vi "Settings for BLE.vi"(0 "Sp_Id_Arr":string[](array[string]), 5 "Ex_Mod_IDs":string[](array[string]), 7 "Est Thresh Val":dbl, 9 "Threshold Value Analysis":bool) -> (4 "Thresh Val":dbl[](array[numeric]), 6 "Index":i32[](array[numeric]), 8 "No of I/ps":i32)   [LabVIEW 2014]
panel:
  in  "Enter Threshold Values":string[][](array[string])=[["GFP", "5", "55", "34"], ["LacI", "10", "55", "34"], ["TetR", "10", "55", "34"]]
  in  "Select Output Specie":u16(ring)=1 items=["GFP", "P1", "P2"]
  in  "OK":bool caption="OK1"
  out "Output Sp":string[](array[string])
  # "Logic Verification Settings"
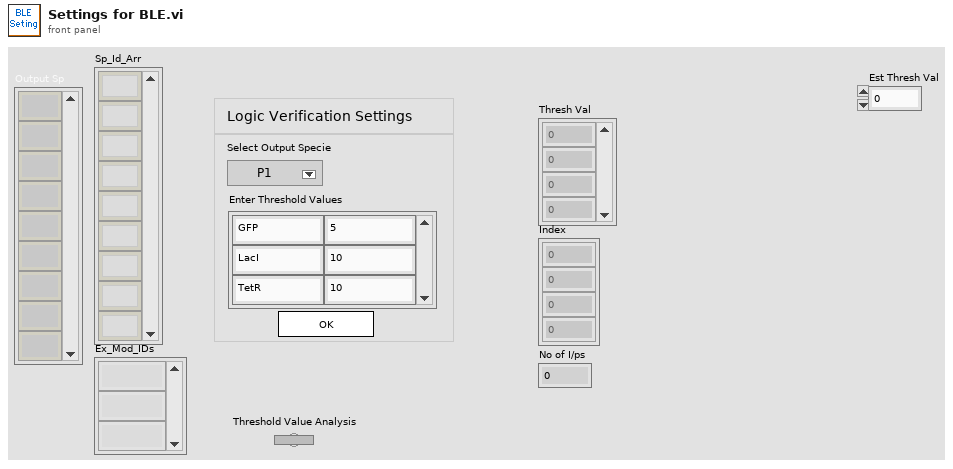
[diagram p1: front panel]
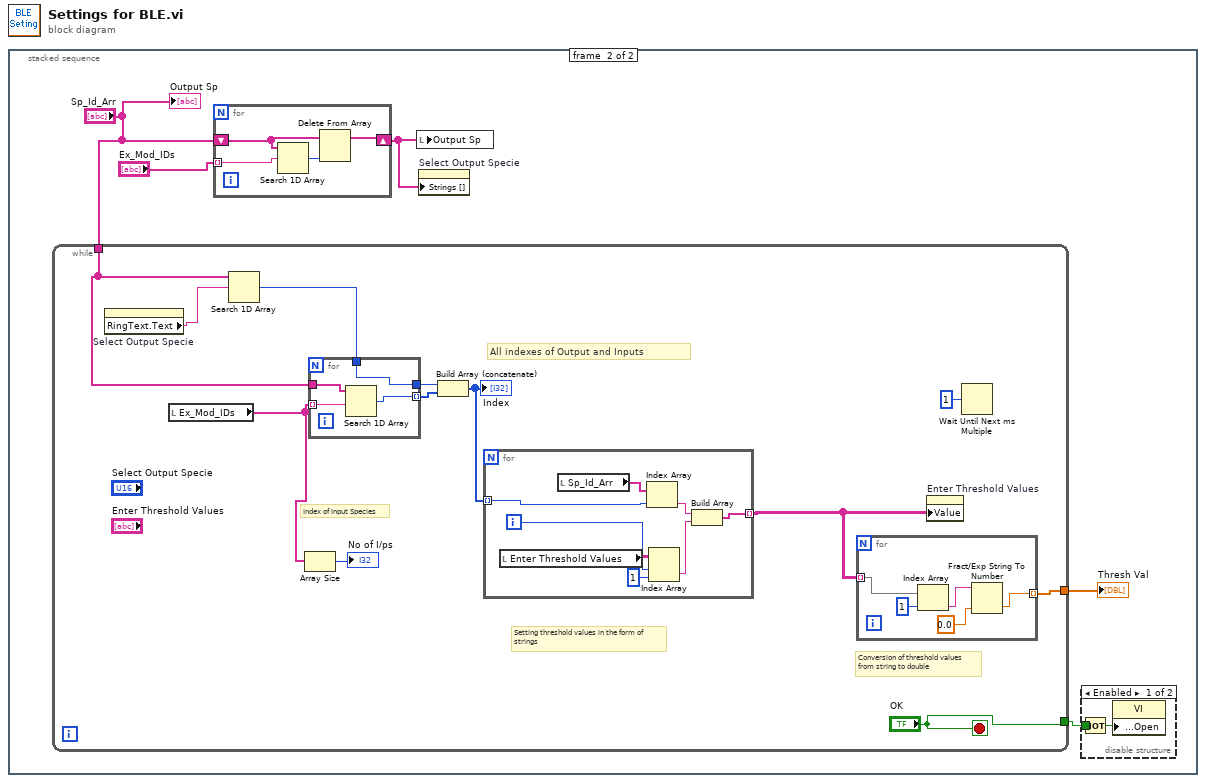
[diagram p0: block diagram]
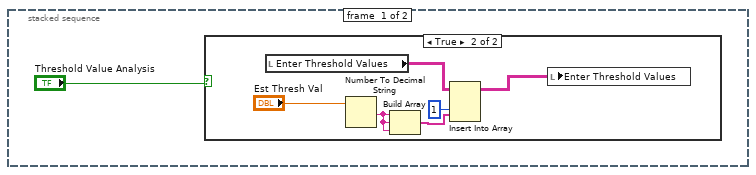
[diagram p2: hidden frame]
diagram:
  n1 = stacked-sequence {
    frame #0 {
      n2 = case shown="True" "Threshold Value Analysis" {
        frame False {
        }
        frame True {
          n3 = local read "Enter Threshold Values"() -> (w7:string[][])
          n4 = Number To Decimal String(number="Est Thresh Val") -> (decimal integer string=w3:string)  [unwired: 1 in]
          n5 = Build Array(w3, w3, w3) -> (w5:string[])
          n6 = Insert Into Array(array=w7, index (col)=1 ("disabled index (col)"), new element=w5) -> (w2:string[][])  [unwired: 1 in]
          n7 = local write "Enter Threshold Values"(w2) -> ()
        }
      }
    }
    frame #1 {
      n8 = while {
        tunnel: "Sp_Id_Arr" -> [w19]
        tunnel: [w18] -> w9
        tunnel: ["OK"] -> w8
        stop <- "OK" stop-if-true
        # "Conversion of threshold values \nfrom string to double"
        # "Setting threshold values in the form of \nstrings"
        # "All indexes of Output and Inputs"
        # "Index of Input Species"
        n9 = property on="Select Output Specie" class="Ring (strict)"() -> ("RingText.Text"=w16:string)  [unwired: 2 in, 2 out]
        n10 = local read "Ex_Mod_IDs"() -> (w25:string[])
        n11 = Search 1D Array(1D array=w19, element=w16) -> (index of element=w20:i32)  [unwired: 1 in]
        n12 = Array Size(array=w25) -> (size(s)=→"No of I/ps":i32)
        n13 = for {
          tunnel: w19 -> [w43]
          tunnel: w25 -> [w42] mode=indexing
          tunnel: [w41] -> w22 mode=indexing
          tunnel: w20 -> [w40]
          tunnel: [w40] -> w21
          n14 = Search 1D Array(1D array=w43, element=w42) -> (index of element=w41:i32)  [unwired: 1 in]
        }
        n15 = Build Array (concatenate)(w21, w22) -> (w23:i32[])
        "Index" <- w23
        n16 = for {
          tunnel: w23 -> [w32] mode=indexing
          tunnel: [w38] -> w24 mode=indexing
          i -> [w34]
          n17 = local read "Enter Threshold Values"() -> (w37:string[][])
          n18 = local read "Sp_Id_Arr"() -> (w39:string[])
          n19 = Index Array(array=w39, index=w32) -> (element=w33:string)
          n20 = Index Array(array=w37, index (row)=w34, index (col)=1 ("disabled index (col)")) -> (element=w35:string)
          n21 = Build Array(w33, w35) -> (w38:string[])
        }
        n22 = for {
          tunnel: w24 -> [w31] mode=indexing
          tunnel: [w28] -> w18 mode=indexing
          n23 = Index Array(array=w31, index=1) -> (element=w29:string)
          n24 = Fract/Exp String To Number(string=w29, default (0 dbl)=0.0) -> (number=w28:dbl)  [unwired: 2 in, 1 out]
        }
        n25 = property on="Enter Threshold Values" class="Arr (strict)"("Value"=w24) -> ()  [unwired: 2 in, 2 out]
        n26 = Wait Until Next ms Multiple(millisecond multiple=u32 1 ("milliseconds to wait")) -> ()  [unwired: 1 out]
      }
      "Thresh Val" <- w9
      n27 = for {
        tunnel: "Ex_Mod_IDs" -> [w46] mode=indexing
        shift-right: [w45] -> w12
        shift-left: "Sp_Id_Arr" -> [w47]
        n28 = Search 1D Array(1D array=w47, element=w46) -> (index of element=w44:i32)  [unwired: 1 in]
        n29 = Delete From Array(array=w47, index=w44) -> (array with subset deleted=w45:string[])  [unwired: 1 in, 1 out]
      }
      n30 = local write "Output Sp"(w12) -> ()
      n31 = property on="Select Output Specie" class="Ring (strict)"("Strings []"=w12) -> ()  [unwired: 2 in, 2 out]
      n32 = disable-structure shown="Enabled" {
        disable-tunnel: w8 -> [w13 _]
        frame Enabled {
          n33 = Not(x=w13) -> (.not. x?=w14:bool)
          n34 = property class="VI"("Front Panel Window:Open"=w14) -> ()  [unwired: 2 in, 2 out]
        }
        frame Disabled {
        }
      }
      "Output Sp" <- "Sp_Id_Arr"
    }
  }
